vi "Check for Idle.vi"(8 "error in (no error)":errorcluster, 9 "Device and Axis":string, 11 "VISA resource name":refnum<visa-resource-name>) -> (0 "error out":errorcluster, 1 "Idle":bool, 3 "VISA resource name out":refnum<visa-resource-name>)   [LabVIEW 2018, in "Zaber A Series.lvlib"]
doc: "Checks whether the device is idle without waiting for it to become idle. To poll a specific device, use the Device and Axis input. This VI is not designed to poll all devices unless only one device is connected.\n\nThis VI requires that the Initialize VI has been called with the same serial port."
uses:
  Zaber A Series.lvlib
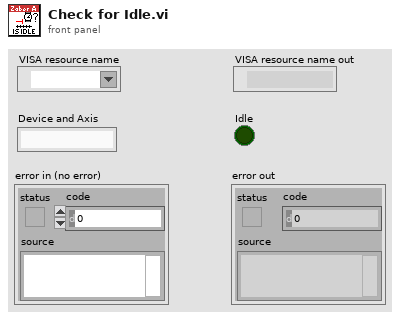
[diagram p1: front panel]
types:
  T1 = cluster{"Device":string, "Axis":string, "Reply Flag":string, "Status":string, "Warning Flags":string, "Data":string}[]
  T2 = cluster{"Device":string, "Axis":string, "Reply Flag":string, "Status":string, "Warning Flags":string, "Data":string}
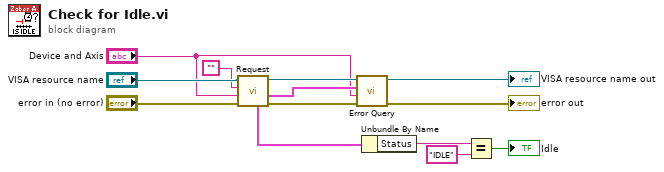
[diagram p0: block diagram]
diagram:
  n1 = call "Request.vi"("error in (no error)"="error in (no error)", "Device and Axis"="Device and Axis", "Command String"="", "VISA resource name"="VISA resource name") -> ("error out"=w6:errorcluster, "Response Bundle Array"=w3:T1, "VISA resource name out"=w7:refnum<visa-resource-name>, "First Response Bundle"=w1:T2)  [unwired: 2 in, 2 out]
  n2 = call "Error Query.vi"("error in (no error)"=w6, "Device and Axis"="Device and Axis", "Previous Response Bundle Array"=w3, "VISA resource name"=w7) -> ("error out"=→"error out":errorcluster, "VISA resource name out"=→"VISA resource name out":refnum<visa-resource-name>)  [unwired: 4 in, 2 out]
  n3 = Unbundle By Name(w1) -> ("Status"=w13:string)
  n4 = Equal?(x=w13, y="IDLE") -> (x = y?=→"Idle":bool)
